vi "Read Child Actor Attributes.vi"(11 "Actor in":refnum<class "Actor.lvclass">) -> (2 "Child Actor Attributes":refnum<data-value>)   [LabVIEW 2020, in "jettl.lvlib" / "Actor.lvclass"]
uses:
  Actor.lvclass
  Child Actor Attributes.ctl
  jettl.lvlib
  Transport/Transport.lvclass
  Actor Attributes.ctl
  Msg/Msg.lvclass
  Msgs.ctl
  Unified Layer.ctl
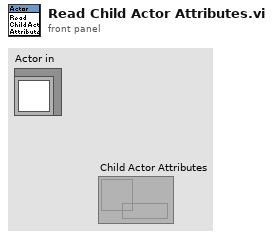
[diagram p1: front panel]
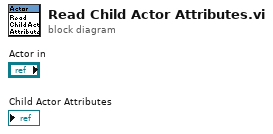
[diagram p0: block diagram]
diagram:
